vi "Write_with_Delay (SubVI).vi"(2 "error in (no error)":errorcluster, 3 "Command":string, 4 "Delay (500ms)":i32=500, 5 "VISA Refnum in":refnum<visa-resource-name>) -> (0 "error out":errorcluster, 1 "VISA Refnum out":refnum<visa-resource-name>)   [LabVIEW 2023]
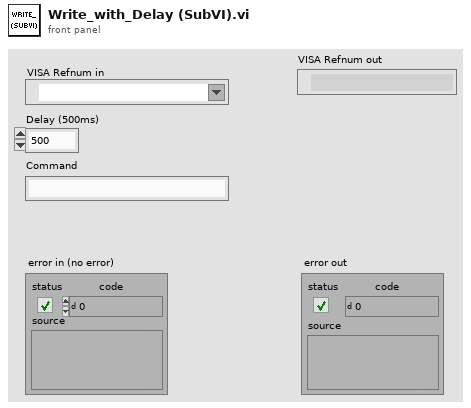
[diagram p1: front panel]
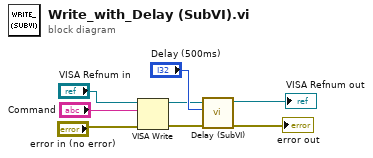
[diagram p0: block diagram]
diagram:
  n1 = VISA Write(VISA resource name="VISA Refnum in", write buffer="Command", error in (no error)="error in (no error)") -> (VISA resource name out=w4:refnum<visa-resource-name>, error out=w5:errorcluster)  [unwired: 1 out]
  n2 = call "Delay (SubVI).vi"("error in (no error)"=w5, "Delay (0 ms)"="Delay (500ms)", "VISA Refnum in"=w4) -> ("error out"=→"error out":errorcluster, "VISA Refnum out"=→"VISA Refnum out":refnum<visa-resource-name>)  [unwired: 7 in]
